vi "AES Get Key & Block Sizes.vi"(8 "error in (no error)":errorcluster) -> (0 "error out":errorcluster, 2 "Block Sizes":i32[](array[numeric]), 3 "Key Sizes":i32[](array[numeric]))   [LabVIEW 2021, in "dotNET Crypto Symmetric Encryption.lvlib"]
uses:
  dotNET Crypto Symmetric Encryption.lvlib
  System.Core
  <vilib>/Analysis/1siggen.llb/Ramp Pattern by Delta.vi
  <vilib>/Analysis/NI_AALBase.lvlib
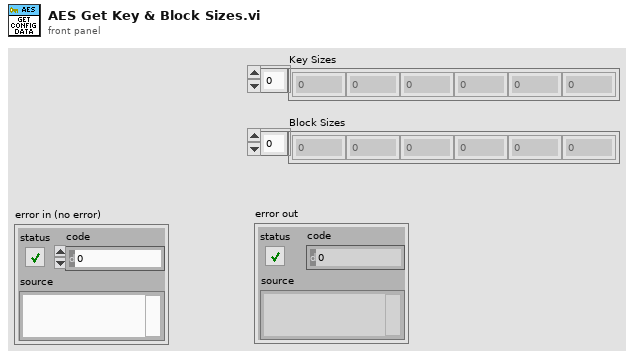
[diagram p1: front panel]
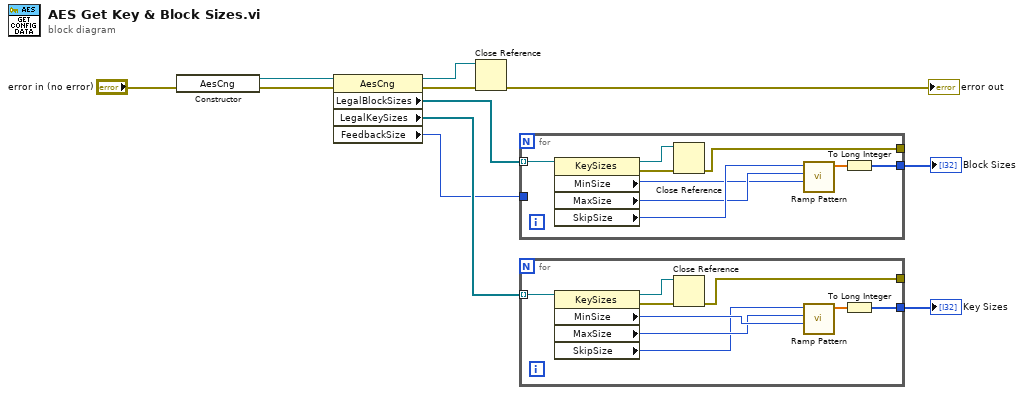
[diagram p0: block diagram]
diagram:
  n1 = constructor class="AesCng"(error in="error in (no error)") -> (reference out=w11:refnum<k24>, error out=w10:errorcluster)  [unwired: 2 in, 1 out]
  n2 = property class="AesCng"(reference=w11, error in=w10) -> (reference out=w8:refnum<k24>, error out=w9:errorcluster, "LegalBlockSizes"=w7:refnum<k24>[], "LegalKeySizes"=w6:refnum<k24>[], "FeedbackSize"=w1:i32)
  n3 = Close Reference(reference=w8, error in (no error)=w9) -> (error out=→"error out":errorcluster)
  n4 = for {
    tunnel: w7 -> [w20] mode=indexing
    tunnel: [w13] -> w4
    tunnel: [w12] -> _
    tunnel: w1 -> [_]
    n5 = property class="KeySizes"(reference=w20) -> (reference out=w18:refnum<k24>, error out=w19:errorcluster, "MinSize"=w14:i32, "MaxSize"=w15:i32, "SkipSize"=w16:i32)  [unwired: 1 in]
    n6 = Close Reference(reference=w18, error in (no error)=w19) -> (error out=w12:errorcluster)
    n7 = call-poly <vilib>:"Ramp Pattern.vi"("start"=w14, "end"=w15, "delta"=w16) -> ("Ramp Pattern"=w17:dbl[])  [unwired: 6 in, 2 out]
    n8 = To Long Integer(number=w17) -> (32bit integer=w13:i32[])
  }
  "Block Sizes" <- w4
  n9 = for {
    tunnel: w6 -> [w29] mode=indexing
    tunnel: [w24] -> w5
    tunnel: [w21] -> _
    n10 = property class="KeySizes"(reference=w29) -> (reference out=w22:refnum<k24>, error out=w23:errorcluster, "MinSize"=w28:i32, "MaxSize"=w27:i32, "SkipSize"=w26:i32)  [unwired: 1 in]
    n11 = Close Reference(reference=w22, error in (no error)=w23) -> (error out=w21:errorcluster)
    n12 = call-poly <vilib>:"Ramp Pattern.vi"("start"=w28, "end"=w27, "delta"=w26) -> ("Ramp Pattern"=w25:dbl[])  [unwired: 6 in, 2 out]
    n13 = To Long Integer(number=w25) -> (32bit integer=w24:i32[])
  }
  "Key Sizes" <- w5
